vi "Dispense.vi"(8 "error in (no error)":errorcluster, 11 "GumballMachine in":refnum<class "GumballMachine.lvclass">) -> (0 "error out":errorcluster, 2 "ProcessMessage":string, 3 "GumballMachine out":refnum<class "GumballMachine.lvclass">)   [LabVIEW 2013, in "GumballMachine.lvclass"]
uses:
  GumballMachine.lvclass
  GumballMachine.lvclass/GumballMachine.ctl
  State.lvclass/State.lvclass
  StateMark.ctl
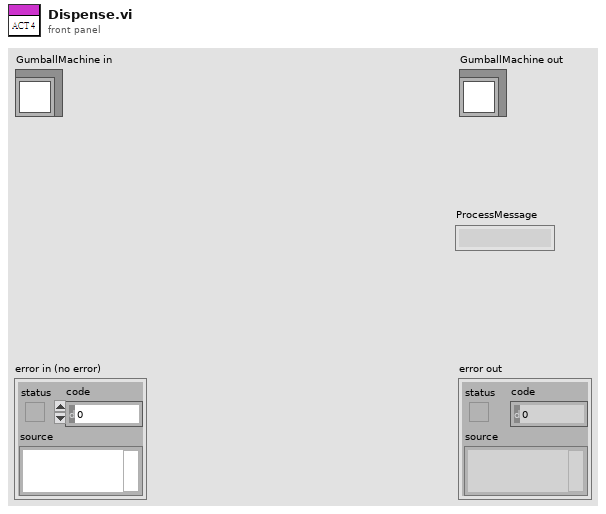
[diagram p1: front panel]
types:
  T1 = typedef "StateMark.ctl" = enum16{"沒有硬幣", "有硬幣", "賣出糖果", "糖果賣完", "NoChange"}
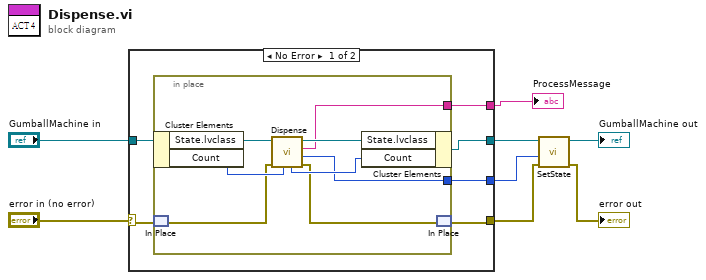
[diagram p0: block diagram]
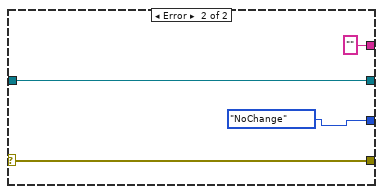
[diagram p2: hidden frame]
diagram:
  n1 = case shown="No Error" "error in (no error)" {
    selector: "error in (no error)" -> [w13 w26]
    tunnel: [w12 w26] -> w3
    tunnel: [w10 w25] -> w5
    tunnel: "GumballMachine in" -> [w14 w25]
    tunnel: [w11 "" ("ProcessMessage")] -> w6
    tunnel: [w9 StateMark."NoChange" ("NextState")] -> w4
    frame No Error {
      n2 = in-place {
        in-place-border: [w20] -> w11
        in-place-border: [w15] -> w9
        n3 = in-place-cluster #1(w14) -> ("State.lvclass"=w22:refnum<class "State.lvclass">, "Count"=w18:i32)
        n4 = in-place-match #2(w13) -> (w17:errorcluster)
        n5 = call-dynamic "Dispense.vi"("Count"=w18, "error in (no error)"=w17, "State in"=w22) -> ("error out"=w16:errorcluster, "NextState"=w15:T1, "ProcessMessage"=w20:string, "State out"=w21:refnum<class "State.lvclass">, "Count Out"=w19:i32)  [unwired: 4 in]
        n6 = in-place-cluster #1("State.lvclass"=w21, "Count"=w19) -> (w10:refnum<class "GumballMachine.lvclass">)
        n7 = in-place-match #2(w16) -> (w12:errorcluster)
      }
    }
    frame Error {
    }
  }
  "ProcessMessage" <- w6
  n8 = call-dynamic "SetState.vi"("error in (no error)"=w3, "State"=w4, "GumballMachine in"=w5) -> ("error out"=→"error out":errorcluster, "GumballMachine out"=→"GumballMachine out":refnum<class "GumballMachine.lvclass">)  [unwired: 7 in]
